vi "Set Shared Variable Refnum.vi"(8 "error in (no error)":errorcluster, 10 "shared variable refnum":refnum<k21>, 11 "abs_SharedVar_Bool in":refnum<class "conc_SharedVar_Var.lvclass">) -> (0 "error out":errorcluster, 3 "abs_SharedVar_Bool out":refnum<class "conc_SharedVar_Var.lvclass">)   [LabVIEW 2021, in "conc_SharedVar_Var.lvclass"]
uses:
  conc_SharedVar_Var.lvclass
  conc_SharedVar_Var.lvclass/conc_SharedVar_Var.ctl
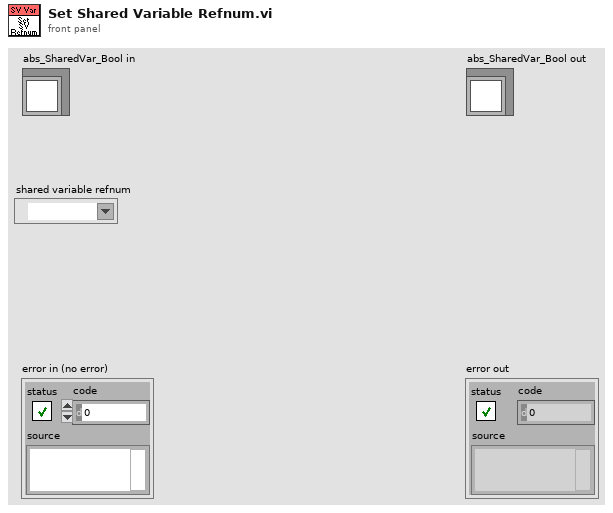
[diagram p1: front panel]
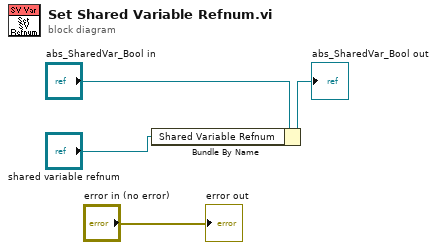
[diagram p0: block diagram]
diagram:
  n1 = Bundle By Name(cluster="abs_SharedVar_Bool in", "Shared Variable Refnum"="shared variable refnum") -> (→"abs_SharedVar_Bool out":refnum<class "conc_SharedVar_Var.lvclass">)
  "error out" <- "error in (no error)"
